vi "WILT Find Water Valve Button.vi"(7 "Search":T1="Water Valve", 10 "Station Number":i32, 11 "Agilent Valve and Switch Locations":T2[](array[typedef])) -> (1 "Station Number":i32, 2 "Agilent Station":string, 3 "Channel":string, 4 "Label":string, 5 "Found Water Valve":bool)   [LabVIEW 2016]
uses:
  Type Definitions/WILT Agilent Channel Definition.ctl
  Type Definitions/WILT Switch Search.ctl
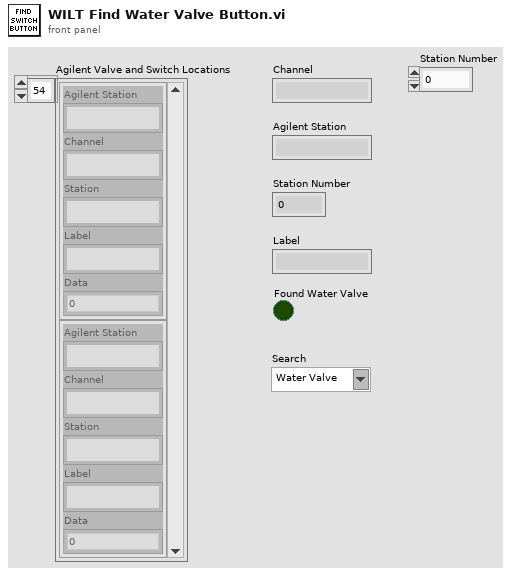
[diagram p1: front panel]
types:
  T1 = typedef "WILT Switch Search.ctl" = string
  T2 = typedef "WILT Agilent Channel Definition.ctl" = cluster{"Channel":string, "Station":string, "Label":string, "Agilent Station":string, "Data":dbl}
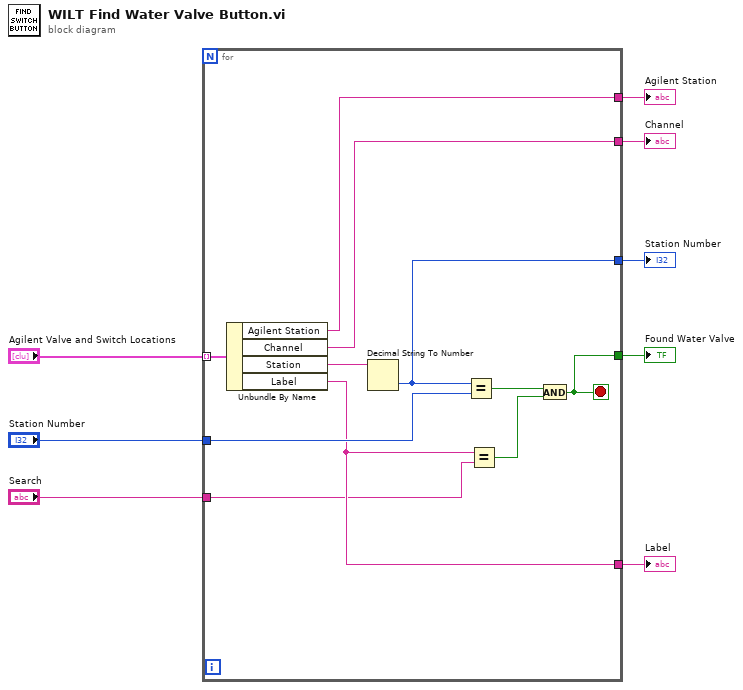
[diagram p0: block diagram]
diagram:
  n1 = for {
    tunnel: "Agilent Valve and Switch Locations" -> [w19] mode=indexing
    tunnel: [w18] -> w6
    tunnel: [w17] -> w5
    tunnel: "Station Number" -> [w15]
    tunnel: [w12] -> w7
    tunnel: [w11] -> w8
    tunnel: [w10] -> w3
    tunnel: "Search" -> [w9]
    stop <- w10 stop-if-true
    n2 = Unbundle By Name(w19) -> ("Agilent Station"=w18:string, "Channel"=w17:string, "Station"=w16:string, "Label"=w11:string)
    n3 = Decimal String To Number(string=w16) -> (number=w12:i32)  [unwired: 2 in, 1 out]
    n4 = Equal?(x=w12, y=w15) -> (x = y?=w13:bool)
    n5 = Equal?(x=w11, y=w9) -> (x = y?=w14:bool)
    n6 = And(x=w13, y=w14) -> (x .and. y?=w10:bool)
  }
  "Label" <- w8
  "Station Number" <- w7
  "Agilent Station" <- w6
  "Channel" <- w5
  "Found Water Valve" <- w3
